vi "LVFunction_Imop_SlopesPostProcessor_Apply PerfectLens.vi"(0 "HasoSlopes in":refnum<class "HasoSlopes.lvclass">, 5 "HasoSlopes OUT":refnum<class "HasoSlopes.lvclass">, 7 "Perfect lens":T1={"lens_m"=0.0, "KeepCurvature"=TRUE}, 11 "error in (no error)":errorcluster) -> (4 "HasoSlopes out":refnum<class "HasoSlopes.lvclass">, 6 "HasoSlopes OUT 2":refnum<class "HasoSlopes.lvclass">, 15 "error out":errorcluster)   [LabVIEW 2020]
doc: "Adds the curvature of a perfect lens to the input slopes.\n\n<B>Slopes_inIn</B> : HasoSlopes object, modified by the processor if Slopes_out = NULL.\n<B>Slopes_inOut</B> : HasoSlopes object, modified by the processor if Slopes_out = NULL.\n<B>focal_lens_m</B> : Perfect lens focal length (m).\n<B>keep_residual_curvature</B> : Keep the residual curvature.\n<B>Slopes_out</B> : processed HasoSlopes object if not NULL."
uses:
  HasoSlopes.lvclass
  SlopesPostProcessorList - Add lens.ctl
  LVClass_HasoSlopes Read HasoSlopes _ property.vi
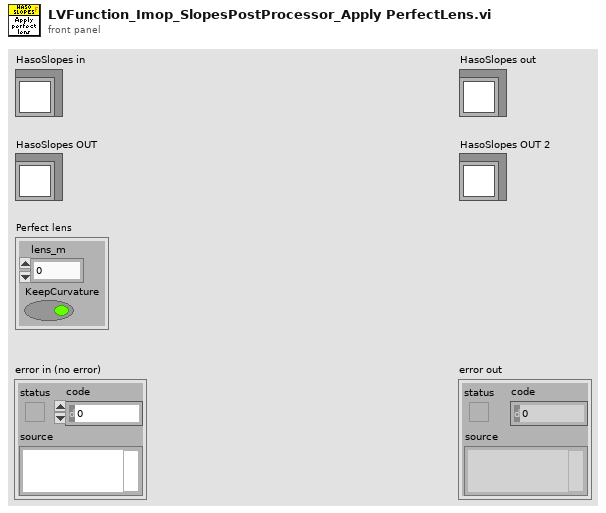
[diagram p1: front panel]
types:
  T1 = typedef "SlopesPostProcessorList - Add lens.ctl" = cluster{"lens_m":sgl, "KeepCurvature":bool}
  T2 = typedef "ClassID.ctl" = i64
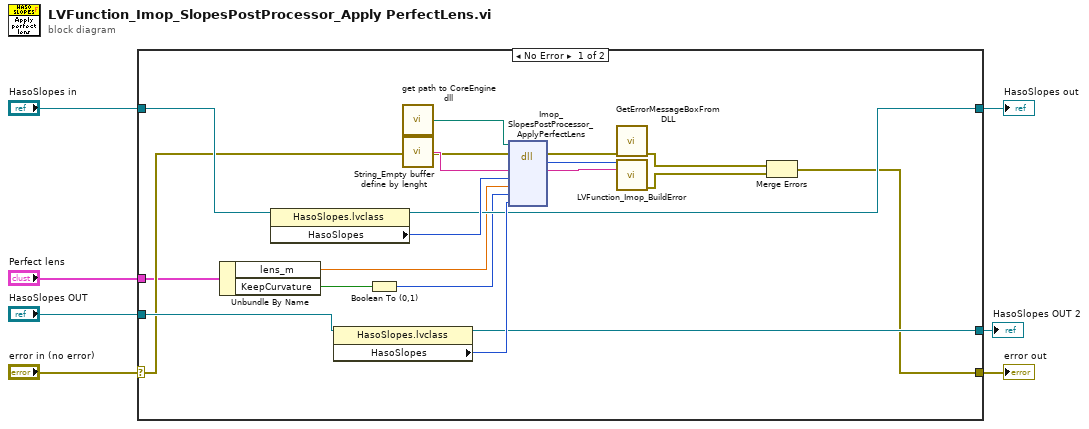
[diagram p0: block diagram]
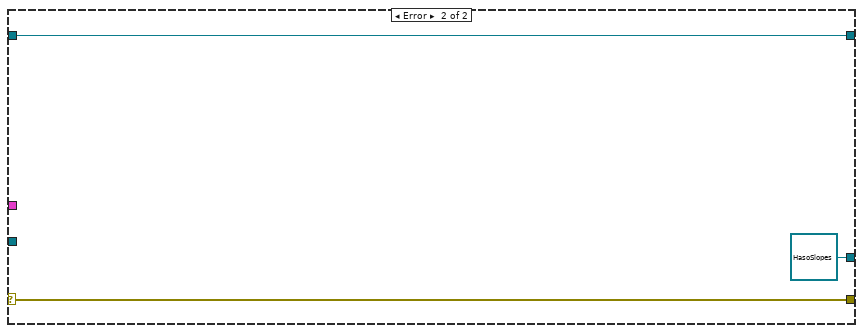
[diagram p2: hidden frame]
diagram:
  n1 = case shown="No Error" "error in (no error)" {
    selector: "error in (no error)" -> [w13 w29]
    tunnel: [w12 w29] -> w6
    tunnel: [w15 w28] -> w4
    tunnel: "HasoSlopes in" -> [w16 w28]
    tunnel: "HasoSlopes OUT" -> [w17 _]
    tunnel: [w14 refnum<class "HasoSlopes.lvclass"> refnum ("HasoSlopes OUT")] -> w2
    tunnel: "Perfect lens" -> [w10 _]
    frame No Error {
      n2 = Unbundle By Name(w10) -> ("lens_m"=w9:sgl, "KeepCurvature"=w8:bool)
      n3 = property class="HasoSlopes.lvclass"(reference=w16) -> (reference out=w15:refnum<class "HasoSlopes.lvclass">, "HasoSlopes"=w26:T2)  [unwired: 1 in, 1 out]
      n4 = property class="HasoSlopes.lvclass"(reference=w17) -> (reference out=w14:refnum<class "HasoSlopes.lvclass">, "HasoSlopes"=w18:T2)  [unwired: 1 in, 1 out]
      n5 = Boolean To (0,1)(Boolean=w8) -> (0, 1=w11:i16)
      n6 = call "get path to CoreEngine dll.vi"() -> ("path to wavekit library"=w21:path)  [unwired: 14 in, 1 out]
      n7 = call "String_Empty buffer define by lenght.vi"() -> ("Empty buffer"=w22:string)  [unwired: 1 in]
      n8 = dll-call lib="D:/FLE/0.Code/CoreEngine4_Suite/LV2011_interface/DLLs/c_interface_vc100.dll" fn="Imop_SlopesPostProcessor_ApplyPerfectLens"(path in=w21, error in=w13, "Message"=w22, "HasoSlopes IN"=w26, "focal  lens m"=w9, "Keep residual curvature"=w11, "HasoSlopes OUT"=w18) -> (error out=w25:errorcluster, "return type"=w23:i32, "Message"=w24:string)  [unwired: 5 in, 1 out]
      n9 = call "GetErrorMessageBoxFromDLL.vi"("error IN"=w25) -> ("error OUT"=w20:errorcluster)  [unwired: 10 in]
      n10 = call "LVFunction_Imop_BuildError.vi"("code"=w23, "String to Prepend to source (\"\")"=w24) -> ("error out"=w19:errorcluster)  [unwired: 13 in]
      n11 = Merge Errors(w20, w19) -> (w12:errorcluster)
    }
    frame Error {
    }
  }
  "error out" <- w6
  "HasoSlopes out" <- w4
  "HasoSlopes OUT 2" <- w2
